vi "DestinationCode.vi"(6 "Single number?":bool=TRUE, 9 "Destination":enum16{"None", "UART", "SPI", "I2C", "WiFi"}(ring), 11 "WiFi Info":T1={"WiFi"={"SSID"="", "Key"=""}, "SystemLink"={"APIKey"="", "Tag"="", "Type"="STRING"}}) -> (1 "Repeated call":string, 2 "Setup":string, 3 "Headers":string)   [LabVIEW 2016]
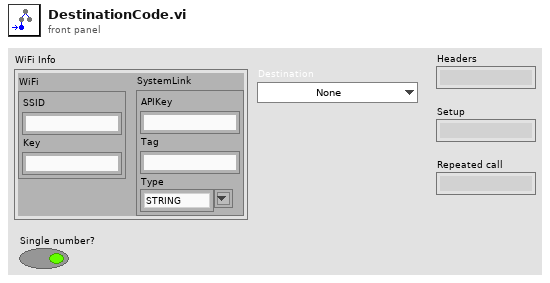
[diagram p1: front panel]
types:
  T1 = cluster{"WiFi":cluster{"SSID":string, "Key":string}, "SystemLink":cluster{"APIKey":string, "Tag":string, "Type":string}}
  T2 = cluster{"APIKey":string, "Tag":string, "Type":string}
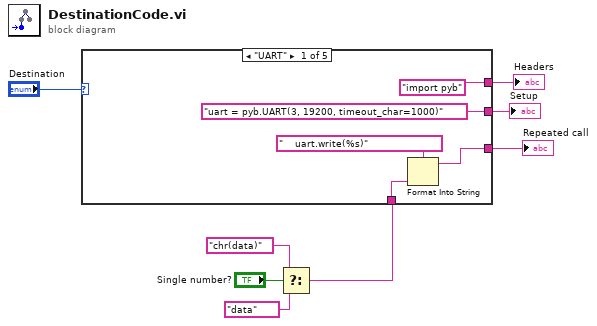
[diagram p0: block diagram]
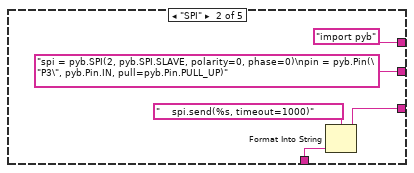
[diagram p2: hidden frame]
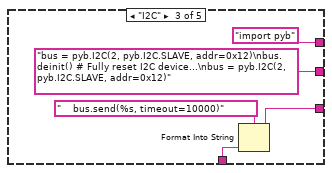
[diagram p3: hidden frame]
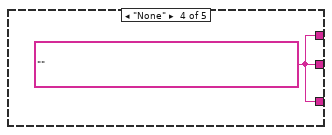
[diagram p4: hidden frame]
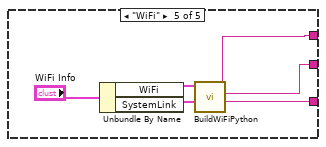
[diagram p5: hidden frame]
diagram:
  n1 = Select(t="chr(data)", s="Single number?", f="data") -> (s? t:f=w3:string)
  n2 = case shown="\"UART\"" "Destination" {
    tunnel: ["uart = pyb.UART(3, 19200, timeout_char=1000)" "spi = pyb.SPI(2, pyb.SPI.SLAVE, polarity=0, phase=0)\npin = pyb.Pin(\"P3\", pyb.Pin.IN, pull=pyb.Pin.PULL_UP)" "bus = pyb.I2C(2, pyb.I2C.SLAVE, addr=0x12)\nbus.deinit() # Fully reset I2C device...\nbus = pyb.I2C(2, pyb.I2C.SLAVE, addr=0x12)" w24 w29] -> w7
    tunnel: [w9 w14 w19 w24 w30] -> w2
    tunnel: ["import pyb" "import pyb" "import pyb" w24 w28] -> w8
    tunnel: w3 -> [w10 w16 w21 _ _]
    frame "UART" {
      n3 = Format Into String(format string="    uart.write(%s)", w10) -> (resulting string=w9:string)  [unwired: 2 in, 1 out]
    }
    frame "SPI" {
      n4 = Format Into String(format string="    spi.send(%s, timeout=1000)", w16) -> (resulting string=w14:string)  [unwired: 2 in, 1 out]
    }
    frame "I2C" {
      n5 = Format Into String(format string="    bus.send(%s, timeout=10000)", w21) -> (resulting string=w19:string)  [unwired: 2 in, 1 out]
    }
    frame "None" {
      w24 = ""
    }
    frame "WiFi" {
      n6 = Unbundle By Name("WiFi Info") -> ("WiFi"=w25:cluster{"SSID":string, "Key":string}, "SystemLink"=w26:T2)
      n7 = call "BuildWiFiPython.vi"("SystemLink"=w26, "WiFi"=w25) -> ("Repeated call"=w30:string, "Setup"=w29:string, "Headers"=w28:string)  [unwired: 7 in]
    }
  }
  "Headers" <- w8
  "Setup" <- w7
  "Repeated call" <- w2
